vi "Configure Frequency Measurement.vi"(7 "Frequency 1 (0: U1)":i32(ring) items=["U1", "I1", "U2", "I2", "U3", "I3", "U4", "I4", "U5", "I5", "U6", "I6"], 8 "error in (no error)":errorcluster, 9 "Frequency 3 (0: U1)":i32(ring) items=["U1", "I1", "U2", "I2", "U3", "I3", "U4", "I4", "U5", "I5", "U6", "I6"], 10 "Frequency 2 (0: U1)":i32(ring) items=["U1", "I1", "U2", "I2", "U3", "I3", "U4", "I4", "U5", "I5", "U6", "I6"], 11 "VISA resource name":refnum<visa-resource-name>) -> (0 "error out":errorcluster, 3 "VISA resource name out":refnum<visa-resource-name>)   [LabVIEW 2021, in "Yokogawa WT1800 Series.lvlib"]
doc: "Configures the frequency measurement features.\n\n<b>Note:</b>\nOn models with the add-on frequency measurement (/FQ) option, \nall input elements can be measured simultaneously, so it is not \nnecessary to use this VI."
uses:
  <instrlib>/Yokogawa WT1800 Series/Yokogawa WT1800 Series.lvlib
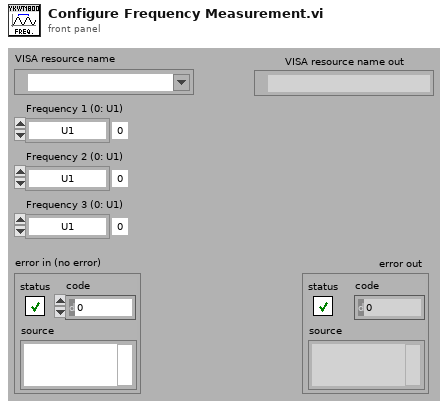
[diagram p1: front panel]
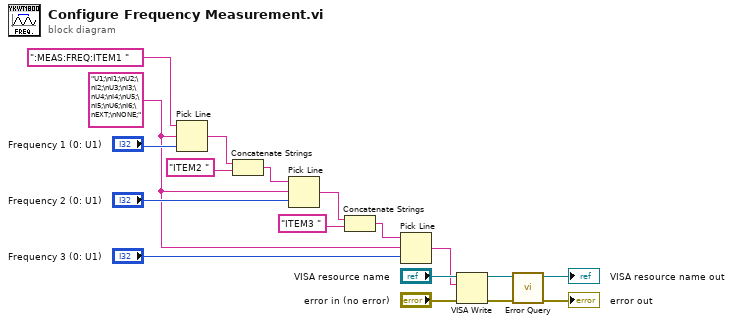
[diagram p0: block diagram]
diagram:
  w3 = "U1;\nI1;\nU2;\nI2;\nU3;\nI3;\nU4;\nI4;\nU5;\nI5;\nU6;\nI6;\nEXT;\nNONE;" ("複数行文字列")
  n1 = Pick Line ("ライン選択")(string ("")=":MEAS:FREQ:ITEM1 ", multi-line string=w3, line index="Frequency 1 (0: U1)") -> (output string=w8:string)
  n2 = Concatenate Strings(w8, "ITEM2 ") -> (w10:string)
  n3 = Pick Line ("ライン選択")(string ("")=w10, multi-line string=w3, line index="Frequency 2 (0: U1)") -> (output string=w4:string)
  n4 = Concatenate Strings(w4, "ITEM3 ") -> (w5:string)
  n5 = Pick Line ("ライン選択")(string ("")=w5, multi-line string=w3, line index="Frequency 3 (0: U1)") -> (output string=w1:string)
  n6 = VISA Write ("VISA書き込み")(VISA resource name="VISA resource name", write buffer=w1, error in (no error)="error in (no error)") -> (VISA resource name out=w18:refnum<visa-resource-name>, error out=w17:errorcluster)  [unwired: 1 out]
  n7 = call <instrlib>:"Error Query.vi"("error in (no error)"=w17, "VISA resource name"=w18) -> ("error out"=→"error out":errorcluster, "VISA resource name out"=→"VISA resource name out":refnum<visa-resource-name>)  [unwired: 6 in, 2 out]
